vi "Instantiate_llm_ollama_embed.vi"(0 "model_name":string(combo), 5 "ollama_url":string="http://localhost:11434/", 11 "error in (no error)":errorcluster) -> (4 "llm_ollama_embedding out":refnum<class "llm_ollama_embedding.lvclass">, 15 "error out":errorcluster)   [LabVIEW 2020, in "llm_ollama_embedding.lvclass"]
uses:
  llm_ollama_embedding.lvclass
  llm_ollama_embedding.lvclass/llm_ollama_embedding.ctl
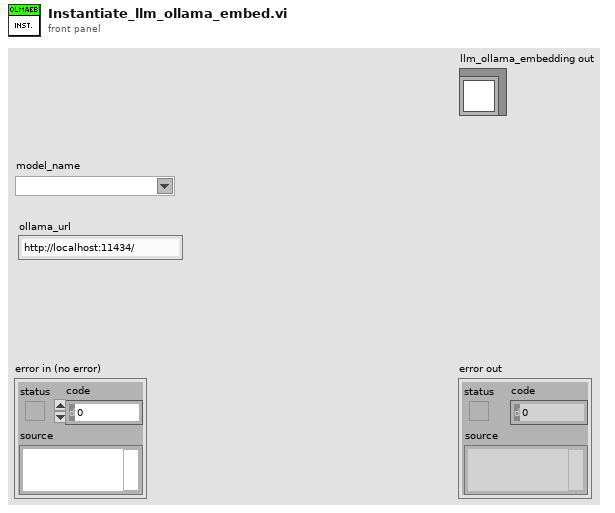
[diagram p1: front panel]
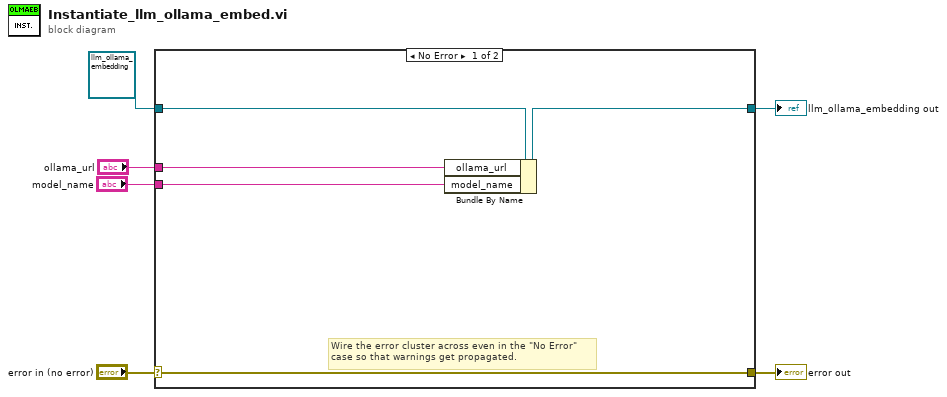
[diagram p0: block diagram]
diagram:
  n1 = case shown="No Error" "error in (no error)" {
    selector: "error in (no error)" -> [w11 w13]
    tunnel: [w11 w13] -> w5
    tunnel: [w8 w12] -> w3
    tunnel: refnum<class "llm_ollama_embedding.lvclass"> refnum ("llm_ollama_embedding in") -> [w10 w12]
    tunnel: "model_name" -> [w9 _]
    tunnel: "ollama_url" -> [w7 _]
    frame No Error {
      # "Wire the error cluster across even in the \"No Error\"\ncase so that warnings get propagated."
      n2 = Bundle By Name(cluster=w10, "ollama_url"=w7, "model_name"=w9) -> (w8:refnum<class "llm_ollama_embedding.lvclass">)
    }
    frame Error {
    }
  }
  "error out" <- w5
  "llm_ollama_embedding out" <- w3
